vi "PostInstall.vi"(10 "Variant":variant) -> (0 "error out":errorcluster)   [LabVIEW 2020]
uses:
  <resource>/dialog/lvconfig.llb/LV Config Read String.vi
  <resource>/dialog/lvconfig.llb/LV Config Write String.vi
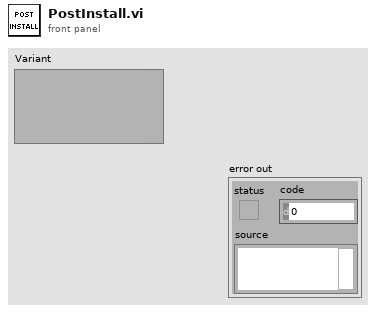
[diagram p1: front panel]
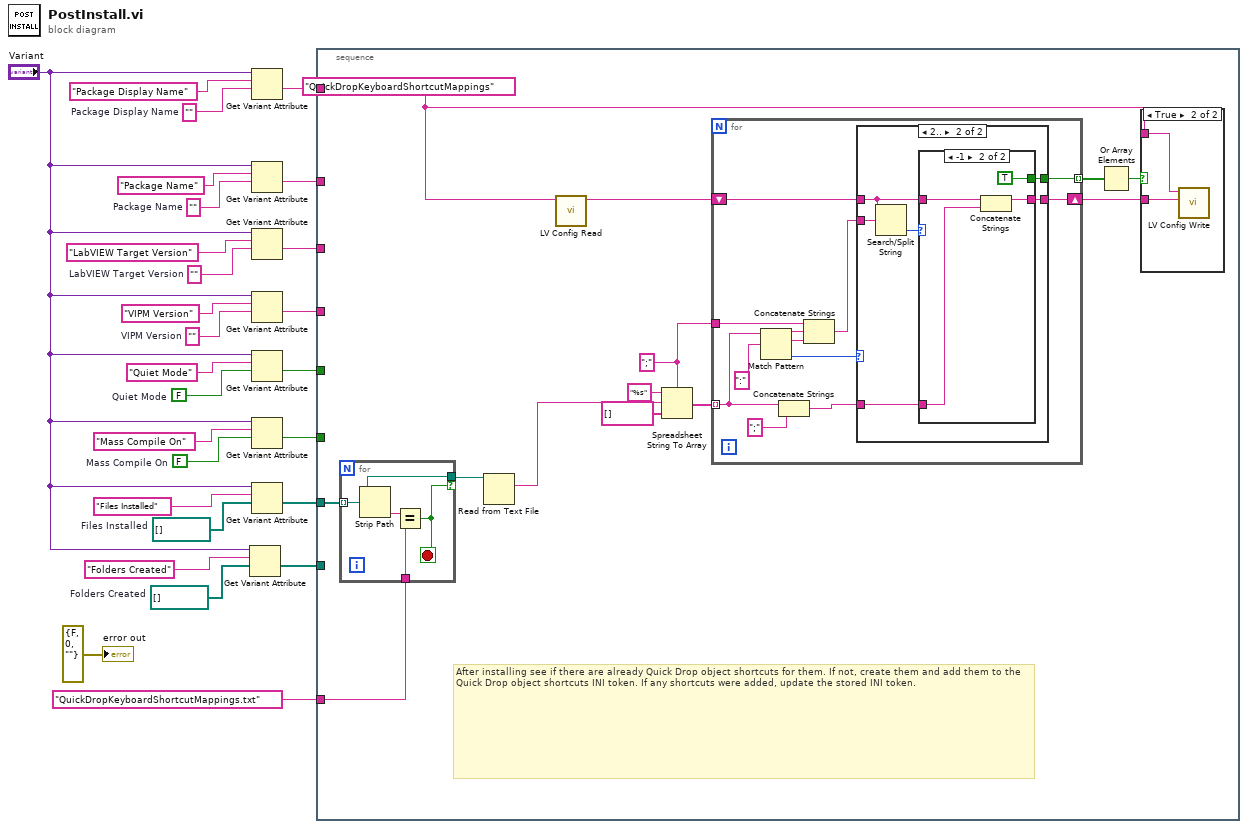
[diagram p0: block diagram]
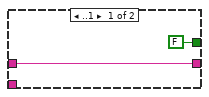
[diagram p2: hidden frame]
diagram:
  w2 = path[] []  # Folders Created
  w3 = path[] []  # Files Installed
  w9 = FALSE  # Mass Compile On
  w10 = ""  # Package Display Name
  w17 = FALSE  # Quiet Mode
  w20 = ""  # VIPM Version
  w22 = ""  # LabVIEW Target Version
  w24 = ""  # Package Name
  n1 = Get Variant Attribute(Variant="Variant", name="Folders Created", default value (empty Variant)=w2) -> (value=w7:path[])  [unwired: 1 in, 3 out]
  n2 = Get Variant Attribute(Variant="Variant", name="Package Display Name", default value (empty Variant)=w10) -> (value=w16:string)  [unwired: 1 in, 3 out]
  n3 = Get Variant Attribute(Variant="Variant", name="Package Name", default value (empty Variant)=w24) -> (value=w15:string)  [unwired: 1 in, 3 out]
  n4 = Get Variant Attribute(Variant="Variant", name="LabVIEW Target Version", default value (empty Variant)=w22) -> (value=w14:string)  [unwired: 1 in, 3 out]
  n5 = Get Variant Attribute(Variant="Variant", name="VIPM Version", default value (empty Variant)=w20) -> (value=w13:string)  [unwired: 1 in, 3 out]
  n6 = Get Variant Attribute(Variant="Variant", name="Quiet Mode", default value (empty Variant)=w17) -> (value=w12:bool)  [unwired: 1 in, 3 out]
  n7 = Get Variant Attribute(Variant="Variant", name="Mass Compile On", default value (empty Variant)=w9) -> (value=w11:bool)  [unwired: 1 in, 3 out]
  n8 = Get Variant Attribute(Variant="Variant", name="Files Installed", default value (empty Variant)=w3) -> (value=w6:path[])  [unwired: 1 in, 3 out]
  n9 = stacked-sequence {
    tunnel: w16 -> [_]
    tunnel: w15 -> [_]
    tunnel: w14 -> [_]
    tunnel: w13 -> [_]
    tunnel: w12 -> [_]
    tunnel: w11 -> [_]
    tunnel: w6 -> [w32]
    tunnel: w7 -> [_]
    tunnel: "QuickDropKeyboardShortcutMappings.txt" ("y") -> [w31]
    frame #0 {
      w28 = ";" ("delimiter (Tab)")
      w40 = "QuickDropKeyboardShortcutMappings" ("key")
      # "After installing see if there are already Quick Drop object shortcuts for them. If not, create them and add them to the Quick Drop object shortcuts INI token. If any shortcuts were added, update the stored INI token."
      n10 = for {
        tunnel: w32 -> [w43] mode=indexing
        tunnel: [w43] -> w30 if=w41
        tunnel: w31 -> [w42]
        stop <- w41 stop-if-true
        n11 = Strip Path(path=w43) -> (name=w44:string)  [unwired: 1 out]
        n12 = Equal?(x=w44, y=w42) -> (x = y?=w41:bool)
      }
      n13 = Read from Text File(file (use dialog)=w30) -> (text=w29:string)  [unwired: 3 in, 3 out]
      n14 = call-poly <resource>:"LV Config Read.vi"("key"=w40) -> ("value"=w39:string)  [unwired: 4 in, 2 out]
      n15 = Spreadsheet String To Array(delimiter (Tab)=w28, format string="%s", spreadsheet string=w29, array type (2D Dbl)=string[] []) -> (array=w33:string[])
      n16 = for {
        shift-right: [w55] -> w36
        shift-left: w39 -> [w56]
        tunnel: w33 -> [w53] mode=indexing
        tunnel: [w54] -> w38 mode=indexing
        tunnel: w28 -> [w49]
        n17 = Match Pattern(string=w53, regular expression=":") -> (before substring=w51:string, match substring=w50:string, offset past match=w47:i32)  [unwired: 1 in, 1 out]
        n18 = Concatenate Strings(w53, ";" ("string")) -> (w46:string)
        n19 = Concatenate Strings(w49, w51, w50) -> (w48:string)
        n20 = case shown="2.." w47 {
          tunnel: w56 -> [w58 w59]
          tunnel: [w58 w63] -> w55
          tunnel: [FALSE w62] -> w54
          tunnel: w46 -> [_ w61]
          tunnel: w48 -> [_ w60]
          frame ..1 {
          }
          frame 2.. {
            n21 = Search/Split String(string=w59, search string/char (-)=w60) -> (offset of match=w64:i32)  [unwired: 1 in, 2 out]
            n22 = case shown="-1" w64 {
              tunnel: w59 -> [w65 w69]
              tunnel: w61 -> [_ w68]
              tunnel: [w65 w67] -> w63
              tunnel: [_ TRUE] -> w62
              frame Default {
              }
              frame -1 {
                n23 = Concatenate Strings(w69, w68) -> (w67:string)
              }
            }
          }
        }
      }
      n24 = Or Array Elements(Boolean array=w38) -> (logical OR=w37:bool)
      n25 = case shown="True" w37 {
        tunnel: w40 -> [_ w71]
        tunnel: w36 -> [_ w70]
        frame False {
        }
        frame True {
          n26 = call-poly <resource>:"LV Config Write.vi"("value"=w70, "key"=w71) -> ()  [unwired: 5 in, 1 out]
        }
      }
    }
  }
  "error out" <- errorcluster {"status"=FALSE, "code"=0, "source"=""} ("error out")
